vi "C. Change Class Control VI Icon.vi"(6 "Variant in":variant, 7 "Shift Pressed?":bool, 8 "error in (no error)":errorcluster, 10 "QD Combo Box Ref":refnum<vi>, 11 "QD Launch VI Ref":refnum<vi>) -> (0 "error out":errorcluster, 4 "Variant out":variant)   [LabVIEW 2020]
doc: "Write a 1-2 sentence description of the functionality of your plugin here. Replace the \"$\" below with the character you wish to assign as the default shortcut for this plugin. Do not add any text after the 'Default Shortcut' line below.\n\nDefault Shortcut - [$]"
uses:
  <vilib>/picture/picture.llb/imagedata.ctl
  <vilib>/Utility/miscctls.llb/LVPoint32TypeDef.ctl
  <vilib>/LabVIEW Icon API/API_User Layer Data.ctl
  <vilib>/LabVIEW Icon API/LabVIEW Icon API.lvlib
panel:
  in  "Undo Name":string="Quick Drop Keyboard Shortcut"
  # "Do not change the connector pane of this VI.\n\nSee the block diagram for directions on how to use this template."
  # "Specify the name of the Undo transaction"
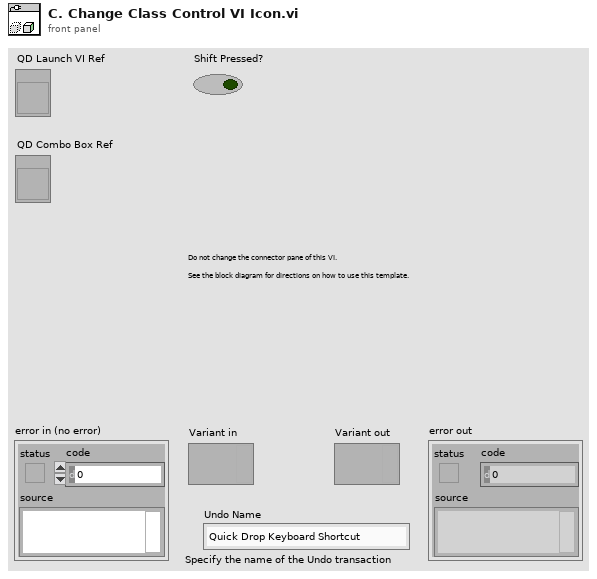
[diagram p1: front panel]
types:
  T1 = enum32{"invalid VI type", "Standard VI", "Control VI", "Global VI", "Polymorphic VI", "Configuration VI", "SubSystem", "Facade VI", "Method VI", "Statechart Diagram VI"}
  T2 = typedef "LVPoint32TypeDef.ctl" = cluster{"Horizontal":i32, "Vertical":i32}
  T3 = typedef "LabVIEW Icon API.lvlib/API_User Layer Data.ctl" = cluster{"Layer name":string, "Origin":T2, "Icon image data":T4}
  T4 = typedef "imagedata.ctl" = cluster{"image type":i32, "image depth":i32, "image":u8[], "mask":u8[], "colors":u32[], "Rectangle":cluster{"left":i16, "top":i16, "right":i16, "bottom":i16}}
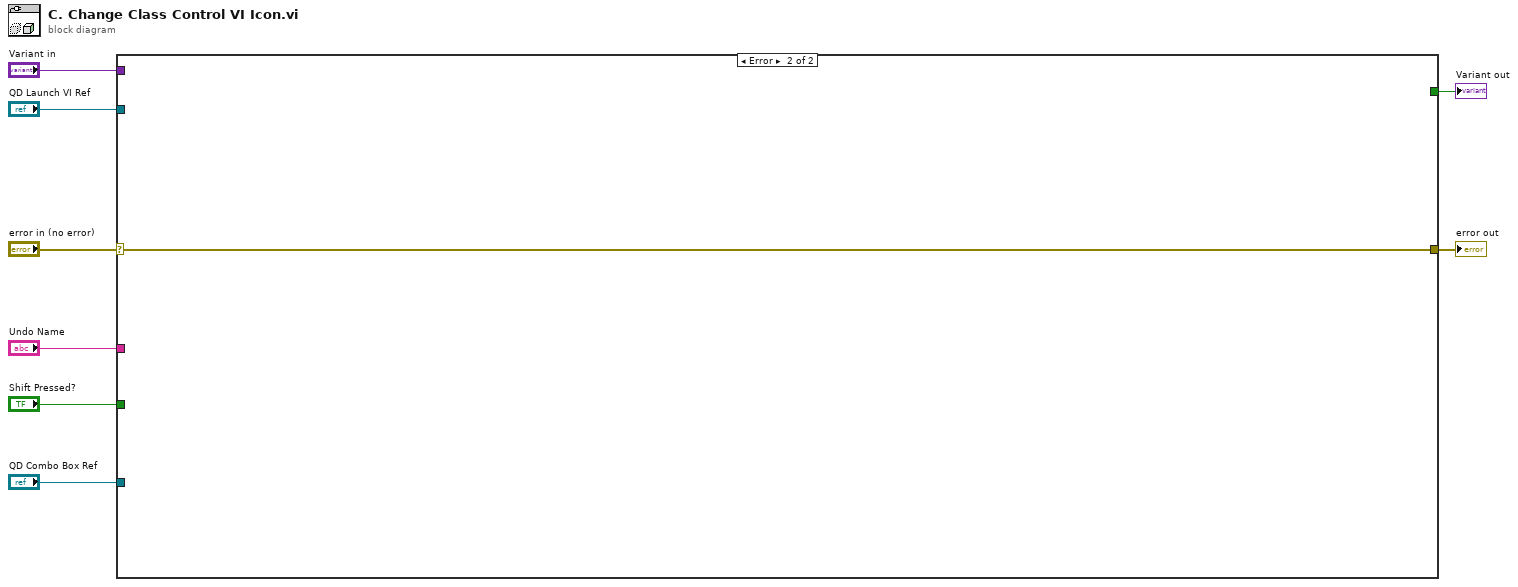
[diagram p0: block diagram]
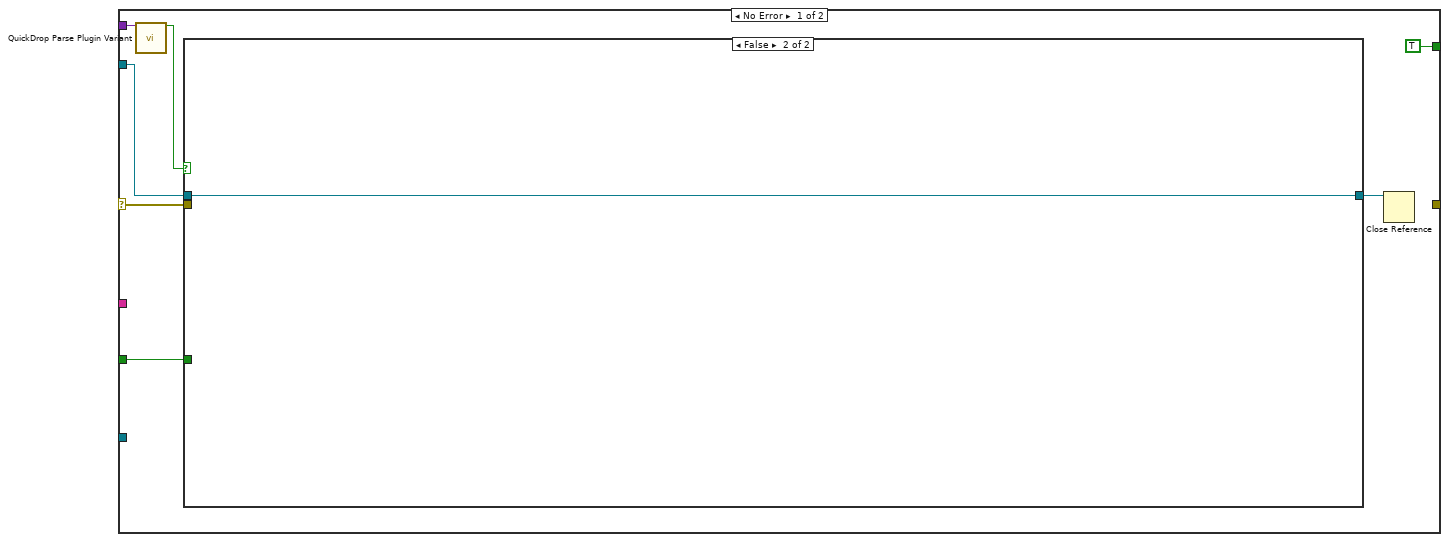
[diagram p2: hidden frame]
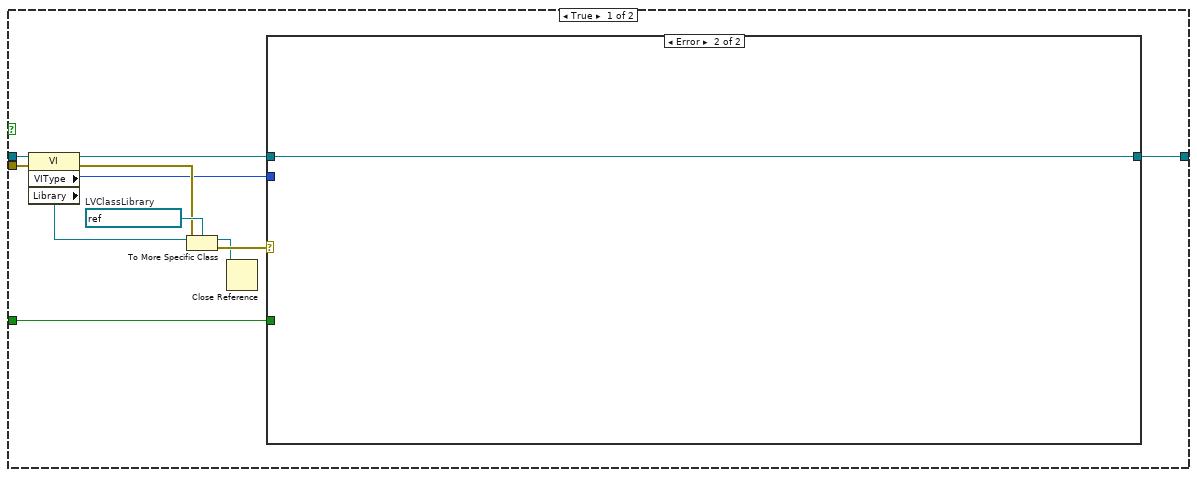
[diagram p3: hidden frame]
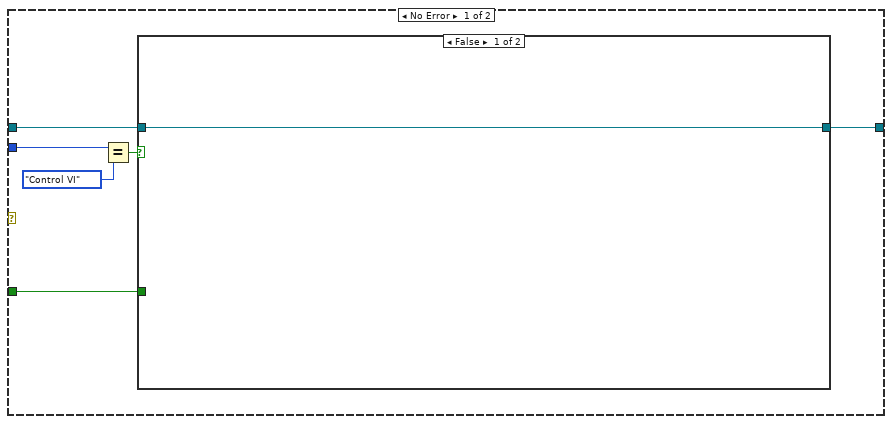
[diagram p4: hidden frame]
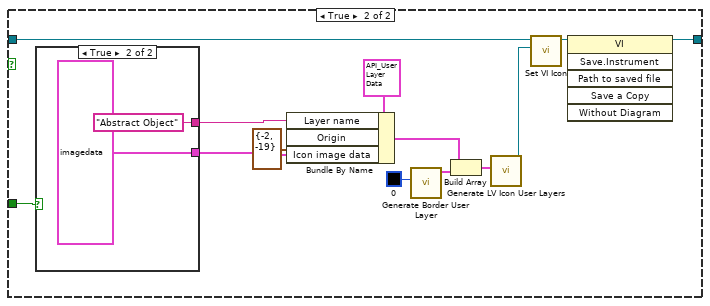
[diagram p5: hidden frame]
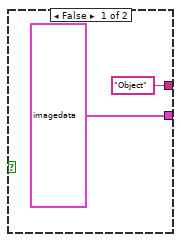
[diagram p6: hidden frame]
diagram:
  n1 = case shown="Error" "error in (no error)" {
    selector: "error in (no error)" -> [w11 w53]
    tunnel: [_ w53] -> w7
    tunnel: "QD Launch VI Ref" -> [w12 _]
    tunnel: "Shift Pressed?" -> [w10 _]
    tunnel: "QD Combo Box Ref" -> [_ _]
    tunnel: "Variant in" -> [w15 _]
    tunnel: "Undo Name" -> [_ _]
    tunnel: [TRUE _] -> w1
    frame No Error {
      n2 = call <vilib>:"QuickDrop Parse Plugin Variant.vi"("QDKS Variant in"=w15) -> ("QD Launch VI Panel?"=w13:bool)  [unwired: 12 in, 2 out]
      n3 = case shown="False" w13 {
        tunnel: w11 -> [w26 _]
        tunnel: w12 -> [w25 w52]
        tunnel: w10 -> [w17 _]
        tunnel: [w16 w52] -> w9
        frame True {
          w24 = refnum<vi> refnum  # LVClassLibrary
          n4 = property class="VI"(reference=w25, error in=w26) -> (reference out=w19:refnum<vi>, error out=w22:errorcluster, "VIType"=w20:T1, "Library"=w23:refnum<vi>)
          n5 = To More Specific Class(target class=w24, reference=w23, error in=w22) -> (specific class reference=w18:refnum<vi>, error out=w21:errorcluster)
          n6 = Close Reference(reference=w18) -> ()  [unwired: 1 in, 1 out]
          n7 = case shown="Error" w21 {
            tunnel: w20 -> [w31 _]
            tunnel: w19 -> [w29 w51]
            tunnel: w17 -> [w28 _]
            tunnel: [w27 w51] -> w16
            frame No Error {
              n8 = Equal?(x=w31, y=T1."Control VI" ("VI Type")) -> (x = y?=w30:bool)
              n9 = case shown="False" w30 {
                tunnel: w29 -> [w33 w46]
                tunnel: w28 -> [_ w34]
                tunnel: [w33 w38] -> w27
                frame False {
                }
                frame True {
                  n10 = case shown="True" w34 {
                    tunnel: ["Object" ("Layer name") "Abstract Object" ("Layer name")] -> w37
                    tunnel: [T4 {"image type"=0, "image depth"=24, "image"=array[3072 elements], "mask"=[], "colors"=[], "Rectangle"={"left"=0, "top"=0, "right"=32, "bottom"=32}} ("Icon image data") T4 {"image type"=0, "image depth"=24, "image"=array[3072 elements], "mask"=[], "colors"=[], "Rectangle"={"left"=0, "top"=0, "right"=32, "bottom"=32}} ("Icon image data")] -> w35
                    frame False {
                    }
                    frame True {
                    }
                  }
                  n11 = Bundle By Name(cluster=T3 {"Layer name"="", "Origin"={"Horizontal"=0, "Vertical"=0}, "Icon image data"={"image type"=0, "image depth"=0, "image"=[], "mask"=[], "colors"=[], "Rectangle"={"left"=0, "top"=0, "right"=0, "bottom"=0}}} ("User layer"), "Layer name"=w37, "Origin"=T2 {"Horizontal"=-2, "Vertical"=-19}, "Icon image data"=w35) -> (w41:T3)
                  n12 = call <vilib>:"Generate Border User Layer.vi"("color(black)"=u32 0) -> ("User Layer data"=w44:T3)  [unwired: 10 in]
                  n13 = Build Array(w41, w44) -> (w43:T3[])
                  n14 = call <vilib>:"Generate LV Icon User Layers.vi"("User layers"=w43) -> ("Icon out"=w40:refnum<class "Icon.lvclass">)  [unwired: 9 in, 1 out]
                  n15 = call <vilib>:"Set VI Icon.vi"("Icon"=w40, "VI Refnum in"=w46) -> ("VI Refnum out"=w39:refnum<vi>)  [unwired: 8 in, 1 out]
                  n16 = invoke class="VI" method="Save.Instrument"(reference=w39) -> (reference out=w38:refnum<vi>)  [unwired: 5 in, 5 out]
                }
              }
            }
            frame Error {
            }
          }
        }
        frame False {
        }
      }
      n17 = Close Reference(reference=w9) -> ()  [unwired: 1 in, 1 out]
    }
    frame Error {
    }
  }
  "error out" <- w7
  "Variant out" <- w1
